vi "getLHeLevel.vi"(8 "error in (no error)":errorcluster, 11 "Instrument.Cryostat in":refnum<class "Instrument.Cryostat.lvclass">) -> (0 "error out":errorcluster, 2 "LHe Level (%)":dbl, 3 "Instrument.Cryostat out":refnum<class "Instrument.Cryostat.lvclass">)   [LabVIEW 2019, in "Instrument.Cryostat.lvclass"]
uses:
  Instrument.Cryostat.lvclass
  C:/Users/patrick/Documents/GitHub/Instrument-Framework/lvsrc/Framework/Instrument/Instrument.lvclass
  Typedefs/Cryostat.commands--enum.ctl
  80e043b3-11a9-4b76-8aa9-8213b4e44572.vi
  80e043b3-11a9-4b76-8aa9-8213b4e44572.vi/8a809b45-0737-4f95-a79f-cb27a37c1a68.vi
  80e043b3-11a9-4b76-8aa9-8213b4e44572.vi/c7e994d5-f1dc-4932-9081-980c82db95dc.vi
  <vilib>/Utility/Data Type/Get Type Information.vi
  <vilib>/JDP Science/JSONtext/JSON text to Variant.vi
  <vilib>/JDP Science/JSONtext/LVClass Serializer/JSONtext LVClass Serializer.lvclass
  Instrument/Instrument.lvclass
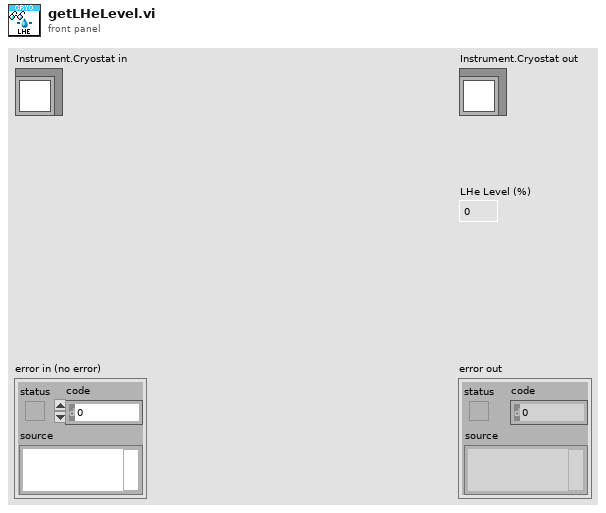
[diagram p1: front panel]
types:
  T1 = typedef "Instrument.Cryostat.lvclass/Cryostat.commands--enum.ctl" = enum16{"getLN2Level", "getLHeLevel", "getMagnet", "getMagnetVector", "setMagnet", "setMagnetVector", "getAngle", "setAngle", "getTemperature", "setTemperature", "getHeater", "setHeater", "getChamber", "setChamber", "getPressure"}
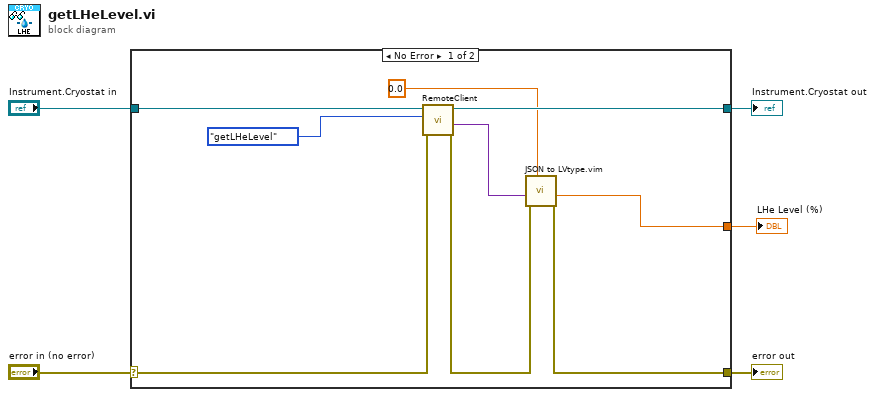
[diagram p0: block diagram]
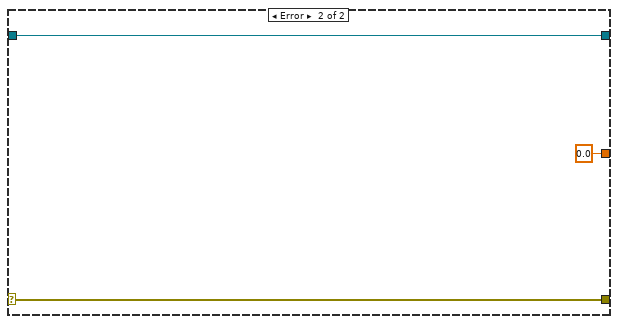
[diagram p2: hidden frame]
diagram:
  n1 = case shown="No Error" "error in (no error)" {
    selector: "error in (no error)" -> [w11 w17]
    tunnel: [w6 w17] -> w4
    tunnel: [w14 w16] -> w2
    tunnel: "Instrument.Cryostat in" -> [w13 w16]
    tunnel: [w7 0.0 ("Data out")] -> w1
    frame No Error {
      n2 = call "RemoteClient.vi"("error in (no error)"=w11, "Command in"=Cryostat.commands--enum."getLHeLevel" ("commands"), "Instrument in"=w13) -> ("error out"=w8:errorcluster, "Data out"=w9:variant, "Instrument out"=w14:refnum<class "Instrument.Cryostat.lvclass">)  [unwired: 5 in, 1 out]
      n3 = call "JSON to LVtype.vim"("type"=0.0, "error in (no error)"=w8, "JSON Data in"=w9) -> ("error out"=w6:errorcluster, "Data out"=w7:dbl)  [unwired: 7 in]
    }
    frame Error {
    }
  }
  "error out" <- w4
  "Instrument.Cryostat out" <- w2
  "LHe Level (%)" <- w1
